vi "RSZVB Get Port Power Offset.vi"(8 "error in (no error)":errorcluster {"code" format="%.0x"}, 9 "Port Number (1)":i32=1, 10 "Channel (1)":i32=1, 11 "VISA session":refnum<visa-resource-name>) -> (0 "error out":errorcluster {"code" format="%.0x"}, 1 "Offset Parameter":i32, 2 "Port Power Offset":dbl format="%^.3e", 3 "dup VISA session":refnum<visa-resource-name>)   [LabVIEW 2011]
doc: "This VI returns a port-specific source power or a power offset relative to the channel power. \n\nRemote-control command(s):\nSOURce<Ch>:POWer<Pt>[:LEVel][:IMMediate]:OFFSet <numeric_value>, ONLY | CPADd"
uses:
  _utility/RSZVB Global Data.vi
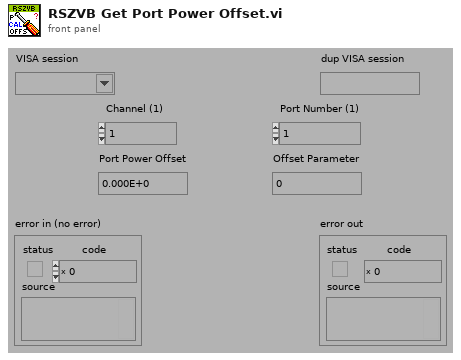
[diagram p1: front panel]
types:
  T1 = cluster{"Error Checking (T: On)":bool, "Installed Options":string[], "Data Valid?":bool, "Ports":i32, "Model":string[], "Option Checking (T: On)":bool}[]
  T2 = cluster{"Error Checking (T: On)":bool, "Installed Options":string[], "Data Valid?":bool, "Ports":i32, "Model":string[], "Option Checking (T: On)":bool}
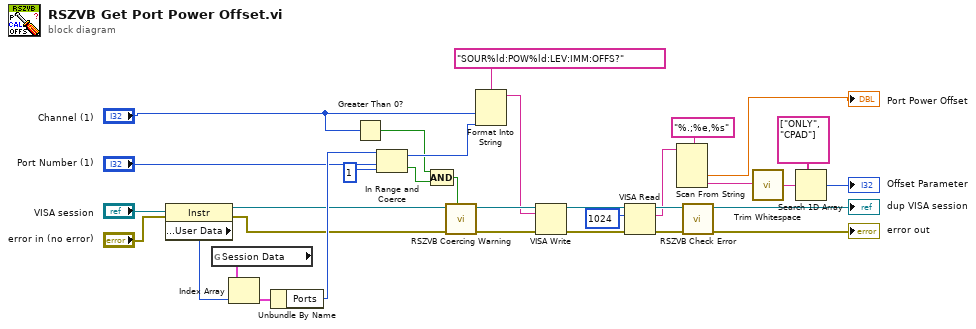
[diagram p0: block diagram]
diagram:
  n1 = property class="Instr"(reference="VISA session", error in="error in (no error)") -> (reference out=w9:refnum<visa-resource-name>, error out=w8:errorcluster, "General Settings:User Data"=w20:u32)
  n2 = global read "RSZVB Global Data.vi" "Session Data"() -> (w21:T1)
  n3 = Index Array(array=w21, index=w20) -> (element=w22:T2)
  n4 = Unbundle By Name(w22) -> ("Ports"=w18:i32)
  n5 = Greater Than 0?(x="Channel (1)") -> (x > 0?=w15:bool)
  n6 = In Range and Coerce(upper limit=w18, x="Port Number (1)", lower limit=1) -> (coerced(x)=w16:i32, In Range?=w14:bool)
  n7 = Compound Arithmetic op=AND(w15, w14) -> (w13:bool)
  n8 = call "RSZVB Coercing Warning.vi"("In Range?"=w13, "error in (no error)"=w8, "VISA session"=w9) -> ("error out"=w25:errorcluster, "dup VISA session"=w26:refnum<visa-resource-name>)  [unwired: 7 in]
  n9 = Format Into String(format string="SOUR%ld:POW%ld:LEV:IMM:OFFS?", "Channel (1)", w16) -> (resulting string=w23:string)  [unwired: 2 in, 1 out]
  n10 = VISA Write(VISA resource name=w26, write buffer=w23, error in (no error)=w25) -> (VISA resource name out=w27:refnum<visa-resource-name>, error out=w28:errorcluster)  [unwired: 1 out]
  n11 = VISA Read(VISA resource name=w27, byte count=u32 1024 ("byte count (0)"), error in (no error)=w28) -> (VISA resource name out=w32:refnum<visa-resource-name>, read buffer=w29:string, error out=w31:errorcluster)  [unwired: 1 out]
  n12 = Scan From String(format string="%.;%e,%s", input string=w29) -> (output 1=→"Port Power Offset":dbl, output 2=w2:string)  [unwired: 4 in, 3 out]
  n13 = call "RSZVB Check Error.vi"("error in (no error)"=w31, "VISA session"=w32) -> ("error out"=→"error out":errorcluster, "dup VISA session"=→"dup VISA session":refnum<visa-resource-name>)  [unwired: 8 in]
  n14 = call <vilib>:"Trim Whitespace.vi"("string"=w2) -> ("trimmed string"=w3:string)  [unwired: 1 in]
  n15 = Search 1D Array(1D array=string[] ["ONLY", "CPAD"] ("array 2"), element=w3) -> (index of element=→"Offset Parameter":i32)  [unwired: 1 in]
